vi "32_filter.vi"() -> ()   [LabVIEW 2018]
uses:
  <vilib>/vision/NI_Vision_Development_Module.lvlib
panel:
  in  "Hue":u8(slide) scale=0.0..255.0
  in  "lower limit":u8(slide)=100 scale=0.0..255.0
  in  "upper limit":u8(slide)=255 scale=0.0..255.0
  out "new":T1(plugin-control)
  out "Array":u8[][](array[numeric])
  out "Image 2":T1(plugin-control)
  out "Image Pixels (U8)":u8[][](array[numeric])
  in  "stop":bool
  out "Image":T1(plugin-control)
  # "Âoªi"
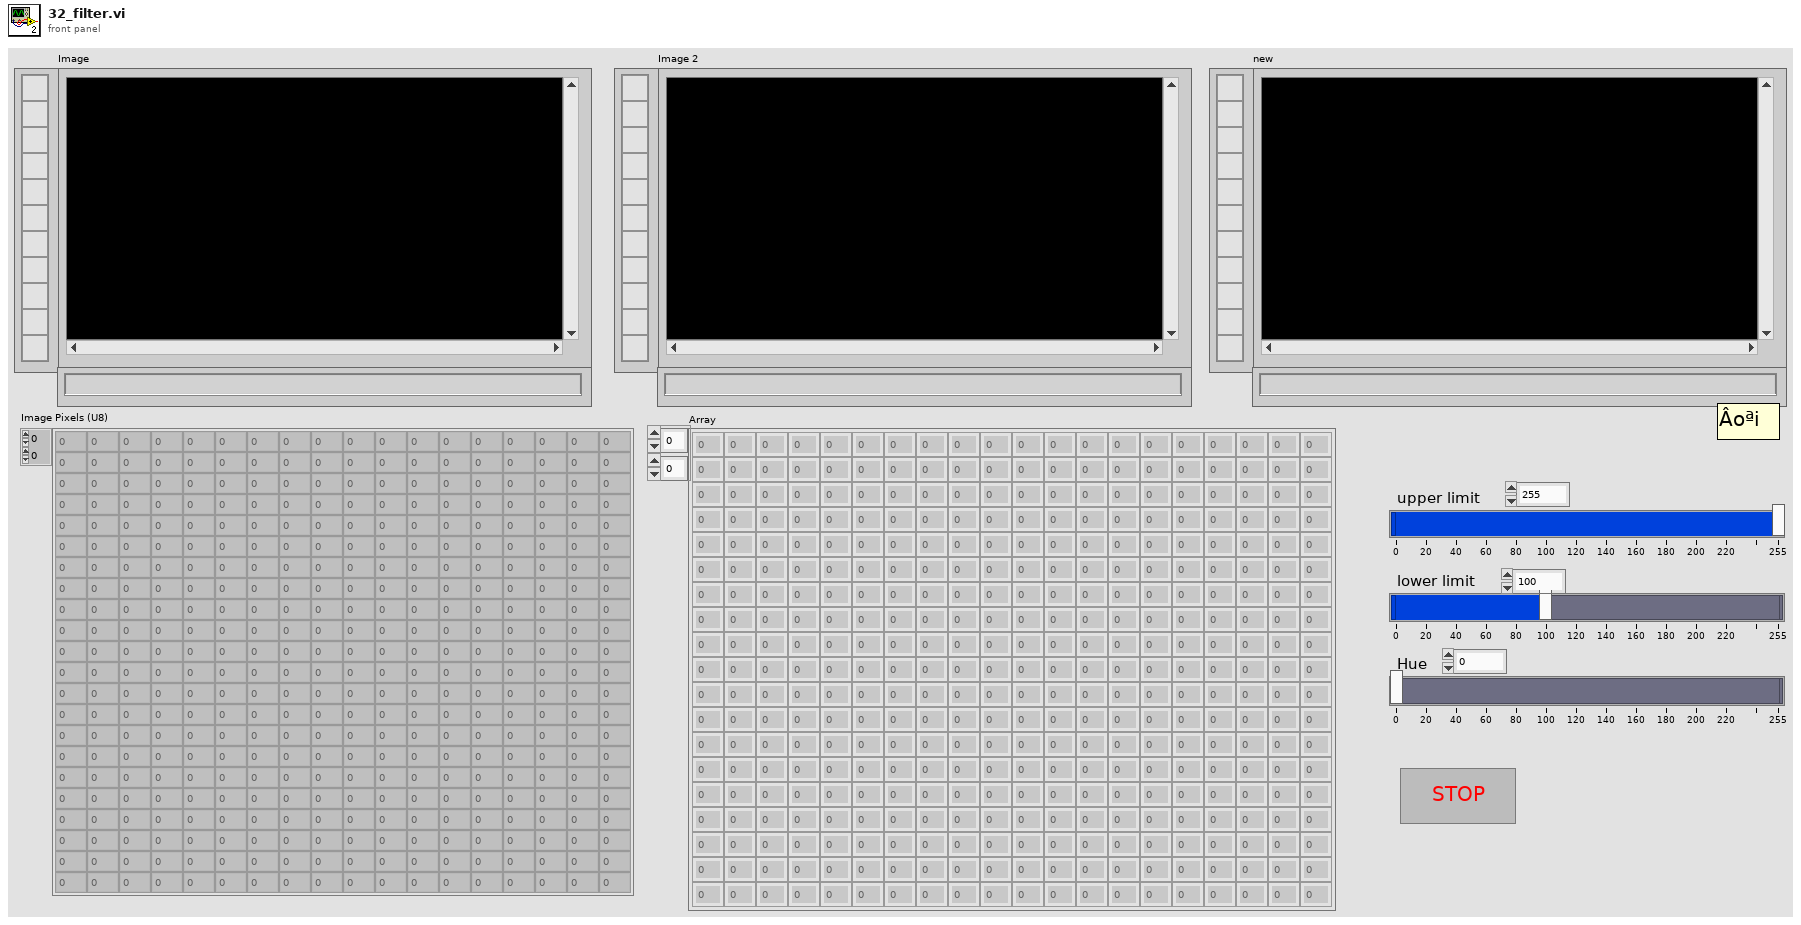
[diagram p1: front panel]
types:
  T1 = typedef "IMAQ Image.ctl" = refnum<image>
  T2 = typedef "Image Type" = u32
  T3 = cluster{"Global Rectangle":i32[], "Contours":cluster{"Contour Type":u32, "ROI Type":u32, "Points":i32[]}[]}
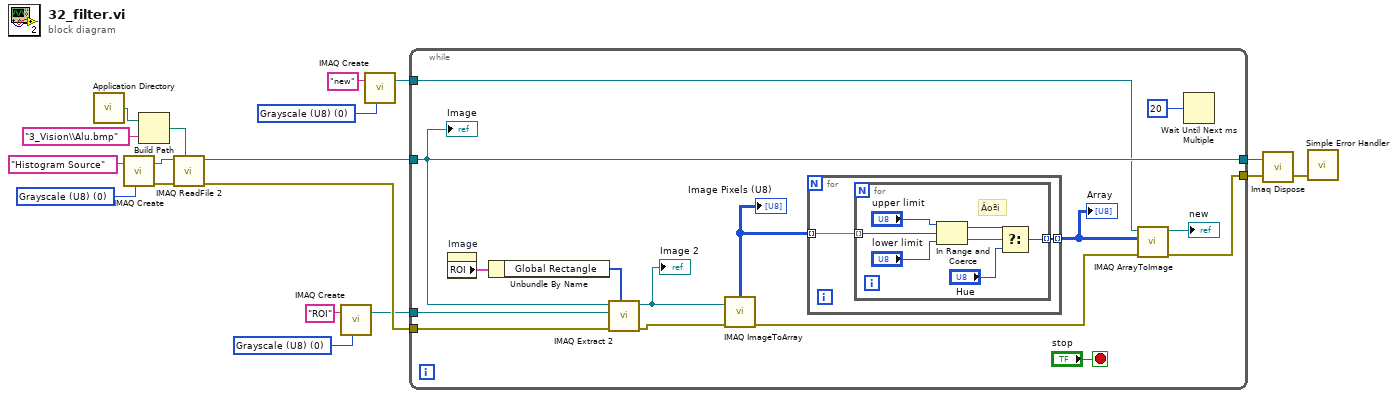
[diagram p0: block diagram]
diagram:
  w2 = T2 0 items=["Grayscale (U8)", "Grayscale (I16)", "Grayscale (SGL)", "Complex (CSG)", "RGB (U32)", "HSL (U32)", "RGB (U64)", "Grayscale (U16)"] ("Image Type")
  w7 = T2 0 items=["Grayscale (U8)", "Grayscale (I16)", "Grayscale (SGL)", "Complex (CSG)", "RGB (U32)", "HSL (U32)", "RGB (U64)", "Grayscale (U16)"] ("Image Type")
  w8 = T2 0 items=["Grayscale (U8)", "Grayscale (I16)", "Grayscale (SGL)", "Complex (CSG)", "RGB (U32)", "HSL (U32)", "RGB (U64)", "Grayscale (U16)"] ("Image Type")
  n1 = call <vilib>:"Application Directory.vi"() -> ("Application Directory"=w10:path)
  n2 = call "IMAQ Create"("Image Name"="Histogram Source", "Image Type"=w8) -> ("New Image"=w18:T1, "error out"=w17:errorcluster)  [unwired: 3 in]
  n3 = Build Path(base path=w10, name or relative path="3_Vision\\Alu.bmp") -> (appended path=w11:path)
  n4 = call "IMAQ ReadFile 2"("File Path"=w11, "error in (no error)"=w17, "Image"=w18) -> ("error out"=w13:errorcluster, "Image Out"=w15:T1)  [unwired: 4 in, 3 out]
  n5 = call "IMAQ Create"("Image Name"="ROI", "Image Type"=w7) -> ("New Image"=w5:T1)  [unwired: 3 in, 1 out]
  n6 = call "IMAQ Create"("Image Name"="new", "Image Type"=w2) -> ("New Image"=w1:T1)  [unwired: 3 in, 1 out]
  n7 = while {
    tunnel: w15 -> [w30]
    tunnel: [w30] -> w14
    tunnel: w13 -> [w27]
    tunnel: w5 -> [w29]
    tunnel: [w19] -> w4
    tunnel: w1 -> [w22]
    stop <- "stop" stop-if-true
    n8 = property on="Image" class="ImageControl"() -> ("ROI"=w31:T3)  [unwired: 2 in, 2 out]
    n9 = Unbundle By Name "Unbundle By Name"(w31) -> ("Global Rectangle"=w28:i32[])
    n10 = call "IMAQ Extract 2"("Optional Rectangle"=w28, "error in (no error)"=w27, "Image Dst"=w29, "Image Src"=w30) -> ("error out"=w25:errorcluster, "Image Dst Out"=w26:T1)  [unwired: 6 in]
    "Image 2" <- w26
    n11 = call "IMAQ ImageToArray"("error in (no error)"=w25, "Image"=w26) -> ("error out"=w20:errorcluster, "Image Pixels (U8)"=w24:u8[][])  [unwired: 2 in, 3 out]
    "Image Pixels (U8)" <- w24
    n12 = for {
      tunnel: w24 -> [w35] mode=indexing
      tunnel: [w34] -> w23 mode=indexing
      n13 = for {
        tunnel: w35 -> [w42] mode=indexing
        tunnel: [w36] -> w34 mode=indexing
        # "Âoªi"
        n14 = In Range and Coerce(upper limit="upper limit", x=w42, lower limit="lower limit") -> (coerced(x)=w38:u8, In Range?=w39:bool)
        n15 = Select(t=w38, s=w39, f="Hue") -> (s? t:f=w36:u8)
      }
    }
    "Array" <- w23
    n16 = call "IMAQ ArrayToImage"("error in (no error)"=w20, "Image Pixels (U8)"=w23, "Image"=w22) -> ("error out"=w19:errorcluster, "Image Out"=→"new":T1)  [unwired: 7 in]
    n17 = Wait Until Next ms Multiple(millisecond multiple=u32 20) -> ()  [unwired: 1 out]
    "Image" <- w30
  }
  n18 = call "Imaq Dispose"("Image"=w14, "error in (no error)"=w4) -> ("error out"=w12:errorcluster)  [unwired: 4 in]
  n19 = call <vilib>:"Simple Error Handler.vi"("error in (no error)"=w12) -> ()  [unwired: 4 in, 5 out]
